vi "BlkHeadWrite.vi"(4 "SequenceOfID":u8[](array[numeric]), 5 "setFileSize":bool=TRUE, 6 "Stimuli":i32, 7 "FramesPerStim":i32, 8 "datatype":u16(ring)=11 items=["U8"=11, "I16"=12, "U32"=13, "SGL"=14], 9 "FrameHeight":i32, 10 "FrameWidth":i32, 11 "引用句柄输入":refnum<file>) -> (3 "引用句柄输出":refnum<file>)   [LabVIEW 2011]
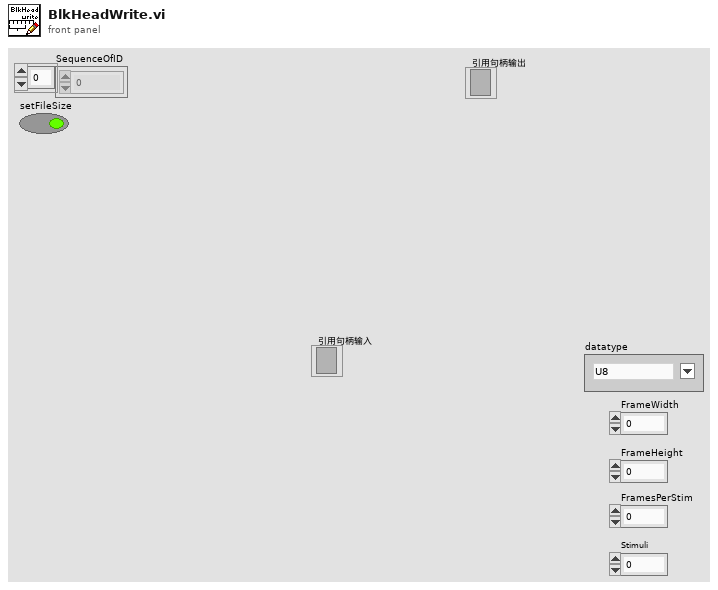
[diagram p1: front panel]
types:
  T1 = enum16{"big-endian, network order", "native, host order", "little-endian"}
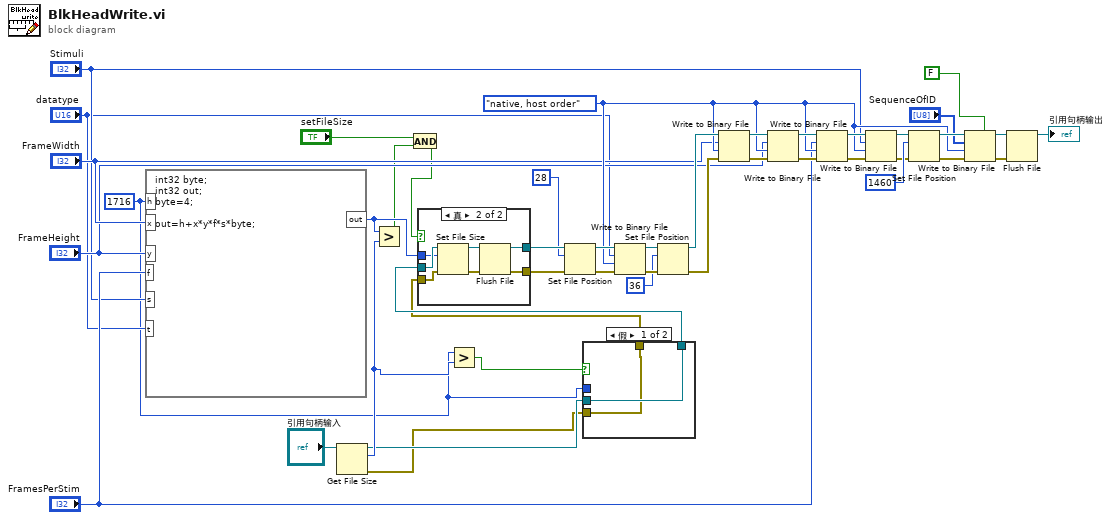
[diagram p0: block diagram]
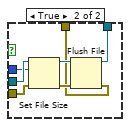
[diagram p2: hidden frame]
diagram:
  w5 = i64 1716 ("大小（字节）")
  w23 = T1."native, host order" ("字节顺序(0:big-endian, network order)")
  n1 = formula code="int32 byte;\nint32 out;\nbyte=4;\n\nout=h+x*y*f*s*byte;"("h"=w5, "x"="FrameWidth", "y"="FrameHeight", "f"="FramesPerStim", "s"="Stimuli", "t"="datatype") -> ("out"=w11:i32)
  n2 = Get File Size(file="引用句柄输入") -> (refnum out=w4:refnum<file>, size (in bytes)=w7:i64, 0:w3:errorcluster)  [unwired: 1 in]
  n3 = Greater?(x=w11, y=w7) -> (0:w9:bool)
  n4 = And(x="setFileSize", y=w9) -> (x .and. y?=w8:bool)
  n5 = Greater?(x=w5, y=w7) -> (0:w6:bool)
  n6 = case shown="假" w6 {
    tunnel: w4 -> [w46 w53]
    tunnel: w3 -> [w45 w52]
    tunnel: w5 -> [_ w51]
    tunnel: [w46 w48] -> w2
    tunnel: [w45 w47] -> w1
    frame False {
    }
    frame True {
      n7 = Set File Size(4:w52, 6:w51, 7:w53) -> (0:w50:errorcluster, 3:w49:refnum<file>)
      n8 = Flush File(refnum=w49, error in=w50) -> (refnum out=w48:refnum<file>, error out=w47:errorcluster)
    }
  }
  n9 = case shown="真" w8 {
    tunnel: [w55 w57] -> w43
    tunnel: w2 -> [w55 w62]
    tunnel: w1 -> [w54 w61]
    tunnel: [w54 w56] -> w42
    tunnel: w11 -> [_ w60]
    frame False {
    }
    frame True {
      n10 = Set File Size(4:w61, 6:w60, 7:w62) -> (0:w59:errorcluster, 3:w58:refnum<file>)
      n11 = Flush File(refnum=w58, error in=w59) -> (refnum out=w57:refnum<file>, error out=w56:errorcluster)
    }
  }
  n12 = Set File Position(offset (in bytes) (0)=i64 28 ("偏移量（字节）（0）"), refnum=w43, error in=w42) -> (refnum out=w44:refnum<file>, error out=w41:errorcluster)  [unwired: 1 in]
  n13 = Write to Binary File(file (use dialog)=w44, data="datatype", error in=w41, 9:w23) -> (refnum out=w38:refnum<file>, error out=w39:errorcluster)  [unwired: 2 in, 1 out]
  n14 = Set File Position(offset (in bytes) (0)=i64 36 ("偏移量（字节）（0）"), refnum=w38, error in=w39) -> (refnum out=w35:refnum<file>, error out=w36:errorcluster)  [unwired: 1 in]
  n15 = Write to Binary File(file (use dialog)=w35, data="FrameWidth", error in=w36, 9:w23) -> (refnum out=w33:refnum<file>, error out=w34:errorcluster)  [unwired: 2 in, 1 out]
  n16 = Write to Binary File(file (use dialog)=w33, data="FrameHeight", error in=w34, 9:w23) -> (refnum out=w31:refnum<file>, error out=w32:errorcluster)  [unwired: 2 in, 1 out]
  n17 = Write to Binary File(file (use dialog)=w31, data="FramesPerStim", error in=w32, 9:w23) -> (refnum out=w30:refnum<file>, error out=w29:errorcluster)  [unwired: 2 in, 1 out]
  n18 = Write to Binary File(file (use dialog)=w30, data="Stimuli", error in=w29, 9:w23) -> (refnum out=w28:refnum<file>, error out=w26:errorcluster)  [unwired: 2 in, 1 out]
  n19 = Set File Position(offset (in bytes) (0)=i64 1460 ("偏移量（字节）（0）"), refnum=w28, error in=w26) -> (refnum out=w25:refnum<file>, error out=w24:errorcluster)  [unwired: 1 in]
  n20 = Write to Binary File(file (use dialog)=w25, data="SequenceOfID", error in=w24, 5:FALSE ("预置数组或字符串大小？(T)"), 9:w23) -> (refnum out=w18:refnum<file>, error out=w19:errorcluster)  [unwired: 1 in, 1 out]
  n21 = Flush File(refnum=w18, error in=w19) -> (refnum out=→"引用句柄输出":refnum<file>)  [unwired: 1 out]
